vi "test_init.vi"() -> ()   [LabVIEW 2020, in "UV-VIS_AVANTES.lvclass"]
uses:
  UV-VIS_AVANTES.lvclass
  C:/dev/TRANCON/Classes/GeneralFunctionality/GeneralFunctionality.lvclass
  C:/dev/TRANCON/Classes/Detector/Detector.lvclass
  Config/Config.lvclass
  UV-VIS_AVANTES.lvclass/UV-VIS_AVANTES.ctl
  GeneralFunctionality/GeneralFunctionality.lvclass/GeneralFunctionality.ctl
  Detector.lvclass/Detector.ctl
  Detector.lvclass
  GeneralFunctionality/GeneralFunctionality.lvclass
panel:
  in  "Path":path=path "C:/Dev/TRANCON/settings/settingsDetector.ini"
  out "error out":errorcluster
  in  "DLL path":path=path "C:/Dev/TRANCON/DLL/avaspec.dll"
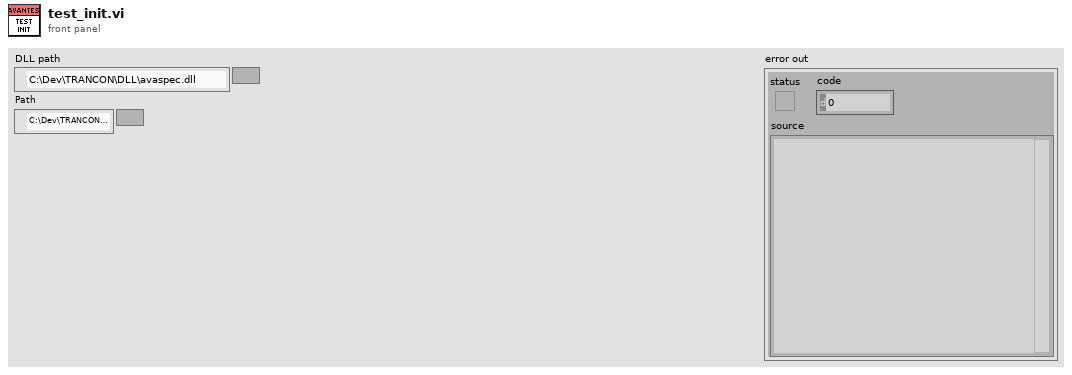
[diagram p1: front panel]
types:
  T1 = typedef "UV-VIS_AVANTES.lvclass/def_parameters.ctl" = cluster{"Len":u16, "ConfigVersion":u16, "UserFriendlyId":u8[], "DetectorType":cluster{"SensorType":u8, "NrPixels":u16, "Fit":sgl[], "NLEnable":u8, "NLCorrect":dbl[], "LowNLCounts":dbl, "HighNLCounts":dbl, "Gain":sgl[], "Reserved":sgl, "Offset":sgl[], "Extern Offset":sgl, "DefectivePixels":u16[]}, "IrradianceType":cluster{"SpectrumCalibrationType":cluster{"SmoothingType":cluster{"m_SmoothPix":u16, "SmoothModel":u8}, "CalInttime":sgl, "CalibConvers":sgl[]}, "CalibrationType":u8, "FiberDiameter":i32}, "SpectrumCalibrationType":cluster{"SmoothingType":cluster{"m_SmoothPix":u16, "SmoothModel":u8}, "CalInttime":sgl, "CalibConvers":sgl[]}, "SpectrumCorrectionType":sgl[], "StandAloneType":cluster{"StandAloneType":u8, "MeasConfigType":cluster{"StartPixel":u16, "StopPixel":u16, "IntegrationTime":sgl, "IntegrationDelay":u32, "NrAverages":u32, "DarkCorrectionType":cluster{"Enable CorDynDark":u8, "ForgetPercentage":u8}, "SmoothingType":cluster{"SmoothPix":u16, "SmoothModel":u8}, "SatDetection":u8, "TriggerType":cluster{"Trigger Mode":u8, "Trigger Source":u8, "Trigger SourceType":u8}, "ControlSettingsType":cluster{"StrobeControl":u16, "LaserDelay":u32, "LaserWidth":u32, "LaserWaveLength":sgl, "StoreToRam":u16}}, "Nmsr":i16}, "DynamicStorageType":cluster{"Nmsr":i32, "Reserved":u8[]}, "TempSensorType":sgl[], "TecControlType":cluster{"Enable":u8, "Setpoint":sgl, "Fit[NR_DAC_POL_COEF]":sgl[]}, "ProcessControlType":cluster{"AnalogLow":sgl[], "AnalogHigh":sgl[], "DigitalLow":sgl[], "DigitalHigh":sgl[]}, "EthernetSettingsType":cluster{"IpAddr":u32, "NetMask":u32, "Gateway":u32, "DhcpEnabled":u8, "TcpPort":u16, "LinkStatus":u8}, "Reserved":u8[]}
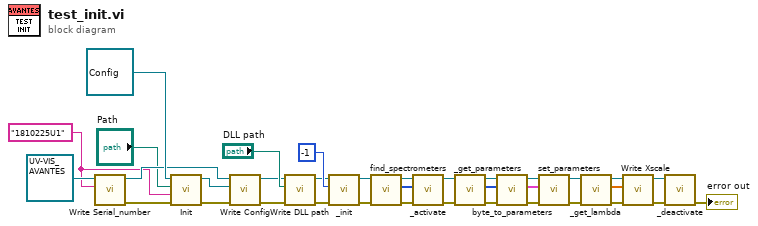
[diagram p0: block diagram]
diagram:
  w1 = "1810225U1" ("Serial_number")
  n1 = call "Write Serial_number.vi"("Serial_number"=w1, "UV-VIS_AVANTES in"=refnum<class "UV-VIS_AVANTES.lvclass"> refnum ("UV-VIS_AVANTES.lvclass")) -> ("error out"=w5:errorcluster, "UV-VIS_AVANTES out"=w8:refnum<class "UV-VIS_AVANTES.lvclass">)  [unwired: 8 in]
  n2 = call "Init.vi"("error in"=w5, "Name"=w1, "Path"="Path", "Config in"=refnum<class "Config.lvclass"> refnum ("Config.lvclass")) -> ("error out"=w4:errorcluster, "Config out"=w6:refnum<class "Config.lvclass">)  [unwired: 6 in]
  n3 = call "Write Config.vi"("error in (no error)"=w4, "Config.lvclass"=w6, "GeneralFunctionality en entrée"=w8) -> ("error out"=w3:errorcluster, "GeneralFunctionality en sortie"=w7:refnum<class "UV-VIS_AVANTES.lvclass">)  [unwired: 7 in]
  n4 = call "Write DLL path.vi"("error in (no error)"=w3, "DLL path"="DLL path", "Detector in"=w7) -> ("error out"=w13:errorcluster, "Detector out"=w14:refnum<class "UV-VIS_AVANTES.lvclass">)  [unwired: 7 in]
  n5 = call "_init.vi"("error in (no error)"=w13, "a_Port"=i16 -1, "UV-VIS_AVANTES in"=w14) -> ("error out"=w33:errorcluster, "UV-VIS_AVANTES out"=w34:refnum<class "UV-VIS_AVANTES.lvclass">)  [unwired: 6 in, 1 out]
  n6 = call "find_spectrometers.vi"("error in (no error)"=w33, "UV-VIS_AVANTES in"=w34) -> ("error out"=w32:errorcluster, "List Output"=w31:u8[], "UV-VIS_AVANTES out"=w35:refnum<class "UV-VIS_AVANTES.lvclass">)  [unwired: 7 in]
  n7 = call "_activate.vi"("error in (no error)"=w32, "a_pDeviceId IN"=w31, "UV-VIS_AVANTES in"=w35) -> ("error out"=w23:errorcluster, "UV-VIS_AVANTES out"=w24:refnum<class "UV-VIS_AVANTES.lvclass">)  [unwired: 7 in]
  n8 = call "_get_parameters.vi"("error in (no error)"=w23, "UV-VIS_AVANTES in"=w24) -> ("error out"=w30:errorcluster, "DeviceParam"=w29:u8[], "UV-VIS_AVANTES out"=w25:refnum<class "UV-VIS_AVANTES.lvclass">)  [unwired: 7 in]
  n9 = call "byte_to_parameters.vi"("error in (no error)"=w30, "DeviceParam"=w29, "UV-VIS_AVANTES in"=w25) -> ("error out"=w26:errorcluster, "parameters cluster"=w28:T1, "UV-VIS_AVANTES out"=w27:refnum<class "UV-VIS_AVANTES.lvclass">)  [unwired: 6 in]
  n10 = call "set_parameters.vi"("error in (no error)"=w26, "AVS_parameters"=w28, "UV-VIS_AVANTES in"=w27) -> ("error out"=w22:errorcluster, "UV-VIS_AVANTES out"=w21:refnum<class "UV-VIS_AVANTES.lvclass">)  [unwired: 7 in]
  n11 = call "_get_lambda.vi"("error in (no error)"=w22, "UV-VIS_AVANTES in"=w21) -> ("error out"=w17:errorcluster, "a_pWaveLength"=w19:dbl[], "UV-VIS_AVANTES out"=w18:refnum<class "UV-VIS_AVANTES.lvclass">)  [unwired: 7 in]
  n12 = call "Write Xscale.vi"("error in (no error)"=w17, "Xscale"=w19, "Detector en entrée"=w18) -> ("error out"=w16:errorcluster, "Detector en sortie"=w15:refnum<class "UV-VIS_AVANTES.lvclass">)  [unwired: 7 in]
  n13 = call "_deactivate.vi"("error in (no error)"=w16, "UV-VIS_AVANTES in"=w15) -> ("error out"=→"error out":errorcluster)  [unwired: 8 in, 1 out]
